vi "ShortcutMenu.vi"(8 "error in":errorcluster, 9 "menu ref in":refnum<k9>, 11 "StepNode in":refnum<class "StepNode.lvclass">) -> (0 "error out":errorcluster, 1 "menu ref out":refnum<k9>, 3 "StepNode out":refnum<class "StepNode.lvclass">)   [LabVIEW 2015, in "StepNode.lvclass"]
doc: "Defines the behavior of the shortcut menu of the node.Copyright 2017 National Instruments Corporation\n\nLicensed under the Apache License, Version 2.0 (the \"License\"); you may not use this file except in compliance with the License. You may obtain a copy of the License at http://www.apache.org/licenses/LICENSE-2.0\nUnless required by applicable law or agreed to in writing, software distributed under the License is distributed on an \"AS IS\" BASIS, WITHOUT WARRANTIES OR CONDITIONS OF ANY KIND, either express or implied. See the License for the specific language governing permissions and limitations under the License."
uses:
  StepNode.lvclass
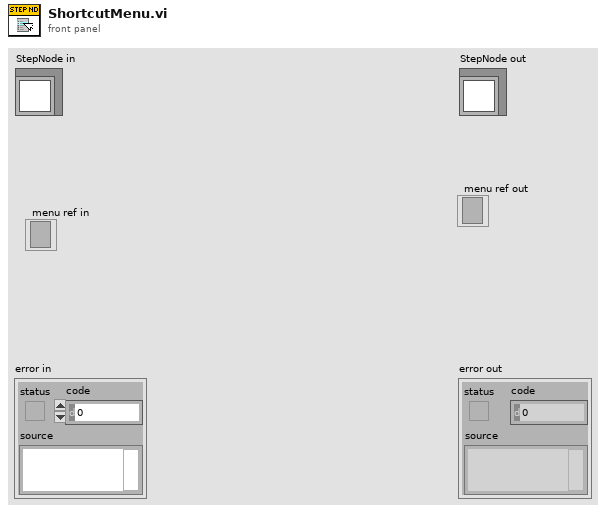
[diagram p1: front panel]
types:
  T1 = typedef "NISE_CEF_Node.lvclass/NodeMenuOptions.ctl" = cluster{"removable":bool, "movable":bool, "duplicate":bool}
  T2 = typedef "NISE_CEF_Node.lvclass/SubNodeCluster.ctl" = cluster{"subnodes menu name":string[], "subnodes class":string[], "subnodes category":string[]}
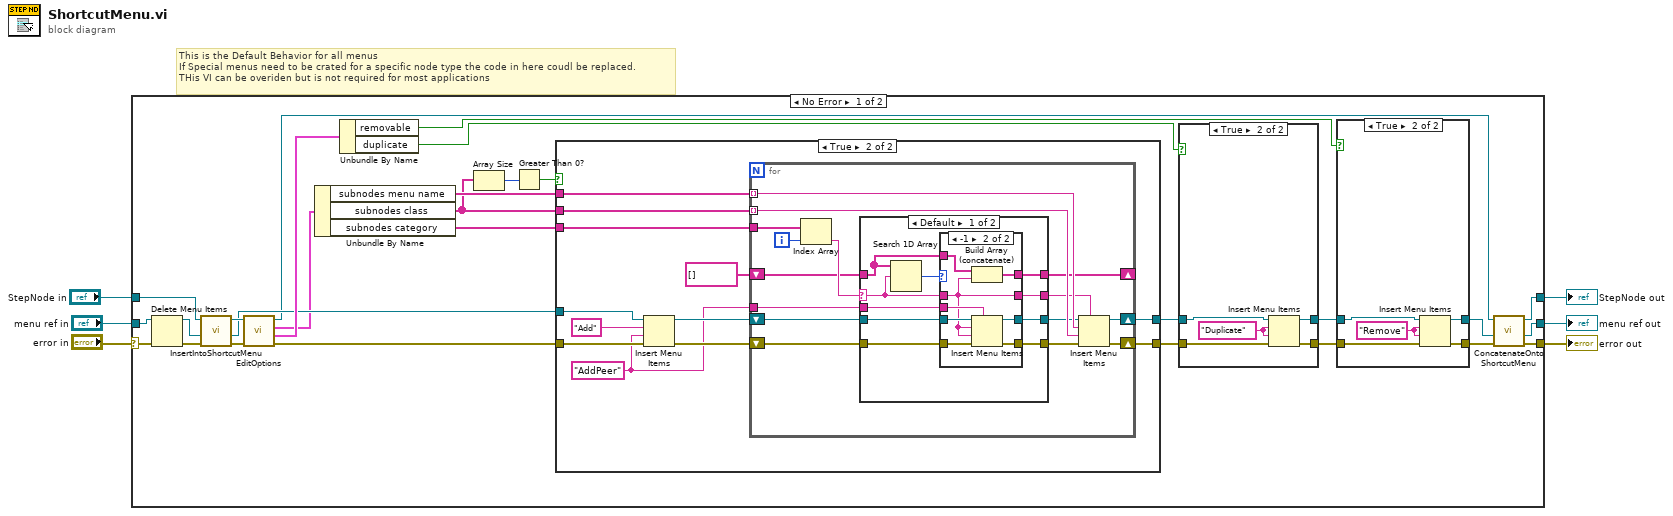
[diagram p0: block diagram]
diagram:
  # "This is the Default Behavior for all menus\nIf Special menus need to be crated for a specific node type the code in here coudl be replaced.\nTHis VI can be overiden but is not required for most applications"
  n1 = case shown="No Error" "error in" {
    selector: "error in" -> [w27 w105]
    tunnel: [w13 w106] -> w3
    tunnel: "StepNode in" -> [w20 w106]
    tunnel: "menu ref in" -> [w30 w104]
    tunnel: [w11 w105] -> w1
    tunnel: [w9 w104] -> w2
    frame No Error {
      n2 = Delete Menu Items(6:w27, 9:w30) -> (0:w18:errorcluster, 3:w21:refnum<k9>)  [unwired: 2 in]
      n3 = call-dynamic "InsertIntoShortcutMenu.vi"("error in"=w18, "menu ref in"=w21, "node in"=w20) -> ("error out"=w17:errorcluster, "menu ref out"=w15:refnum<k9>, "node out"=w19:refnum<class "StepNode.lvclass">)  [unwired: 6 in]
      n4 = call-dynamic "EditOptions.vi"("error in"=w17, "channel in"=w19) -> ("error out"=w16:errorcluster, "edit options"=w29:T1, "subnodes class"=w8:T2, "channel out"=w14:refnum<class "StepNode.lvclass">)  [unwired: 6 in]
      n5 = Unbundle By Name(w8) -> ("subnodes menu name"=w23:string[], "subnodes class"=w22:string[], "subnodes category"=w7:string[])
      n6 = Unbundle By Name(w29) -> ("removable"=w24:bool, "duplicate"=w28:bool)
      n7 = Array Size(array=w22) -> (size(s)=w34:i32)
      n8 = Greater Than 0?(x=w34) -> (x > 0?=w33:bool)
      n9 = case shown="True" w33 {
        tunnel: w15 -> [w50 w62]
        tunnel: w16 -> [w49 w61]
        tunnel: w23 -> [_ w58]
        tunnel: [w50 w57] -> w32
        tunnel: [w49 w56] -> w31
        tunnel: w22 -> [_ w55]
        tunnel: w7 -> [_ w53]
        frame False {
        }
        frame True {
          w51 = "AddPeer"
          n10 = Insert Menu Items(6:w61, 7:w51, 8:"Add", 9:w62) -> (0:w59:errorcluster, 3:w60:refnum<k9>)  [unwired: 2 in, 1 out]
          n11 = for {
            tunnel: w51 -> [w69]
            tunnel: w58 -> [w75] mode=indexing
            shift-right: [w77] -> w57
            shift-left: w60 -> [w66]
            shift-right: [w76] -> w56
            shift-left: w59 -> [w64]
            tunnel: w55 -> [w74] mode=indexing
            tunnel: w53 -> [w73]
            shift-right: [w67] -> _
            shift-left: string[] [] -> [w68]
            i -> [w72]
            n12 = Index Array(array=w73, index=w72) -> (element=w71:string)
            n13 = case shown="Default" w71 {
              selector: w71 -> [w85 _]
              tunnel: [w86 w103] -> w70
              tunnel: w69 -> [w80 w103]
              tunnel: w68 -> [w84 w102]
              tunnel: [w83 w102] -> w67
              tunnel: w66 -> [w82 w101]
              tunnel: [w81 w101] -> w65
              tunnel: w64 -> [w79 w100]
              tunnel: [w78 w100] -> w63
              frame Default {
                n14 = Search 1D Array(1D array=w84, element=w85) -> (index of element=w87:i32)  [unwired: 1 in]
                n15 = case shown="-1" w87 {
                  tunnel: [w89 w94] -> w86
                  tunnel: w85 -> [w89 w94]
                  tunnel: w84 -> [w90 w99]
                  tunnel: [w90 w98] -> w83
                  tunnel: w82 -> [w91 w97]
                  tunnel: [w91 w96] -> w81
                  tunnel: w80 -> [_ w95]
                  tunnel: w79 -> [w88 w93]
                  tunnel: [w88 w92] -> w78
                  frame Default {
                  }
                  frame -1 {
                    n16 = Build Array (concatenate)(w99, w94) -> (w98:string[])
                    n17 = Insert Menu Items(5:w95, 6:w93, 7:w94, 8:w94, 9:w97) -> (0:w92:errorcluster, 3:w96:refnum<k9>)  [unwired: 1 in, 1 out]
                  }
                }
              }
              frame "" {
              }
            }
            n18 = Insert Menu Items(5:w70, 6:w63, 7:w74, 8:w75, 9:w65) -> (0:w76:errorcluster, 3:w77:refnum<k9>)  [unwired: 1 in, 1 out]
          }
        }
      }
      n19 = case shown="True" w28 {
        tunnel: w32 -> [w43 w48]
        tunnel: w31 -> [w42 w47]
        tunnel: [w43 w46] -> w25
        tunnel: [w42 w45] -> w26
        frame False {
        }
        frame True {
          w44 = "Duplicate"
          n20 = Insert Menu Items(6:w47, 7:w44, 8:w44, 9:w48) -> (0:w45:errorcluster, 3:w46:refnum<k9>)  [unwired: 2 in, 1 out]
        }
      }
      n21 = case shown="True" w24 {
        tunnel: w26 -> [w36 w41]
        tunnel: [w36 w40] -> w12
        tunnel: w25 -> [w35 w39]
        tunnel: [w35 w38] -> w10
        frame False {
        }
        frame True {
          w37 = "Remove"
          n22 = Insert Menu Items(6:w41, 7:w37, 8:w37, 9:w39) -> (0:w40:errorcluster, 3:w38:refnum<k9>)  [unwired: 2 in, 1 out]
        }
      }
      n23 = call-dynamic "ConcatenateOntoShortcutMenu.vi"("error in"=w12, "menu ref in"=w10, "node in"=w14) -> ("error out"=w11:errorcluster, "menu ref out"=w9:refnum<k9>, "node out"=w13:refnum<class "StepNode.lvclass">)  [unwired: 6 in]
    }
    frame Error {
    }
  }
  "error out" <- w1
  "StepNode out" <- w3
  "menu ref out" <- w2
